vi "makeSelectTransactionsQueryTemplate.vi"() -> (3 "SELECT Query":string)   [LabVIEW 2018, in "Account History.lvclass"]
uses:
  Account History.lvclass
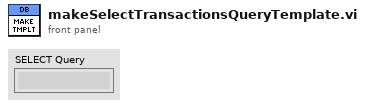
[diagram p1: front panel]
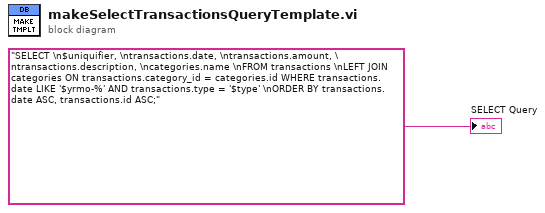
[diagram p0: block diagram]
diagram:
  "SELECT Query" <- "SELECT \n$uniquifier, \ntransactions.date, \ntransactions.amount, \ntransactions.description, \ncategories.name \nFROM transactions \nLEFT JOIN categories ON transactions.category_id = categories.id WHERE transactions.date LIKE '$yrmo-%' AND transactions.type = '$type' \nORDER BY transactions.date ASC, transactions.id ASC;"
